vi "Main_UI_AutoPaste_2.vi"(8 "error in (no error)":errorcluster) -> (0 "error out":errorcluster)   [LabVIEW 2019]
uses:
  <vilib>/Utility/miscctls.llb/LVPointTypeDef.ctl
  <vilib>/Utility/miscctls.llb/LVPositionTypeDef.ctl
  Ctrl/Auto Inspection Main UI Ref.ctl
  Ctrl/tray icon.ctl
  Ctrl/Table Save.ctl
  Ctrl/Auto Inspection Station Name2.ctl
  Ctrl/Auto Inspection Data Name.ctl
  Function/Main UI/Glb/Main_UI Gb.vi
  Global/Process Global.vi
  LLB/Commonly VI.lvlib
panel:
  in  "NG Pick finish":bool
  in  "NG Pick arrive":bool
  in  "AI finish":bool
  in  "AI arrive":bool
  in  "LineScanfinish":bool
  in  "LineScan arrive":bool
  out "Station Name 3":string="Pick"
  in  "TrayStatus":u32[][](array[colorbox])
  in  "Tab Control":enum32{"UI", "AI  image"}(tab)
  out "Laser Station 2":string="S11 Laser Point Station"
  out "Barcode Station 2":string="S1 Barcode Station"
  out "S4 Tool String Display":string="Barcode Station"
  out "Station Name 5":string="Table4"
  out "電流":string="S4 T2 電流"
  out "電壓":string="S2 T1 電壓"
  out "Laser Station":string="Laser Point Station"
  out "Station Name 4":string="Table3"
  out "Station Name 1":string="Table1"
  out "Station Name 2":string="Table2"
  out "Barcode Status":string
  out "Laser Status":string
  out "T2 buffer":string
  out "Laser Data 2":string="S11雷射量測值"
  out "Laser Data":dbl
  out "T1 Current00":dbl
  out "S2 Tool String Display":string="Barcode Station"
  out "S3Tool String Display":string="Barcode Station"
  out "Boolean 2":bool
  out "Boolean 3":bool
  out "Boolean 4":bool
  out "Boolean 5":bool
  out "Boolean 6":bool
  out "Boolean 7":bool
  out "S2Initial":bool
  out "S2Format":bool
  out "S2Program":bool
  out "S2Scan":bool
  out "S2Reset":bool
  out "S2 T1":bool
  out "S3Initial":bool
  out "S3Format":bool
  out "S3Program":bool
  out "S3Scan":bool
  out "S3Reset":bool
  out "S3 T":bool
  out "S4Initial":bool
  out "S4Format":bool
  out "S4Program":bool
  out "S4Scan":bool
  out "S4Reset":bool
  out "S4 T":bool
  out "Total Table 2":cluster{"Table Control":string[][]}[](array[cluster])
  out "EnfMeasureTable":cluster{"Table Control":string[][]}[](array[cluster])
  out "Vision AI Status":string
  out "S8 Vision AI":string="S8 Vision AI"
  out "Barcode Action":string="Barcode Action"
  out "Vision AI":string="Barcode Action"
  out "Image 2":T1(plugin-control)
  out "image":T1(plugin-control)
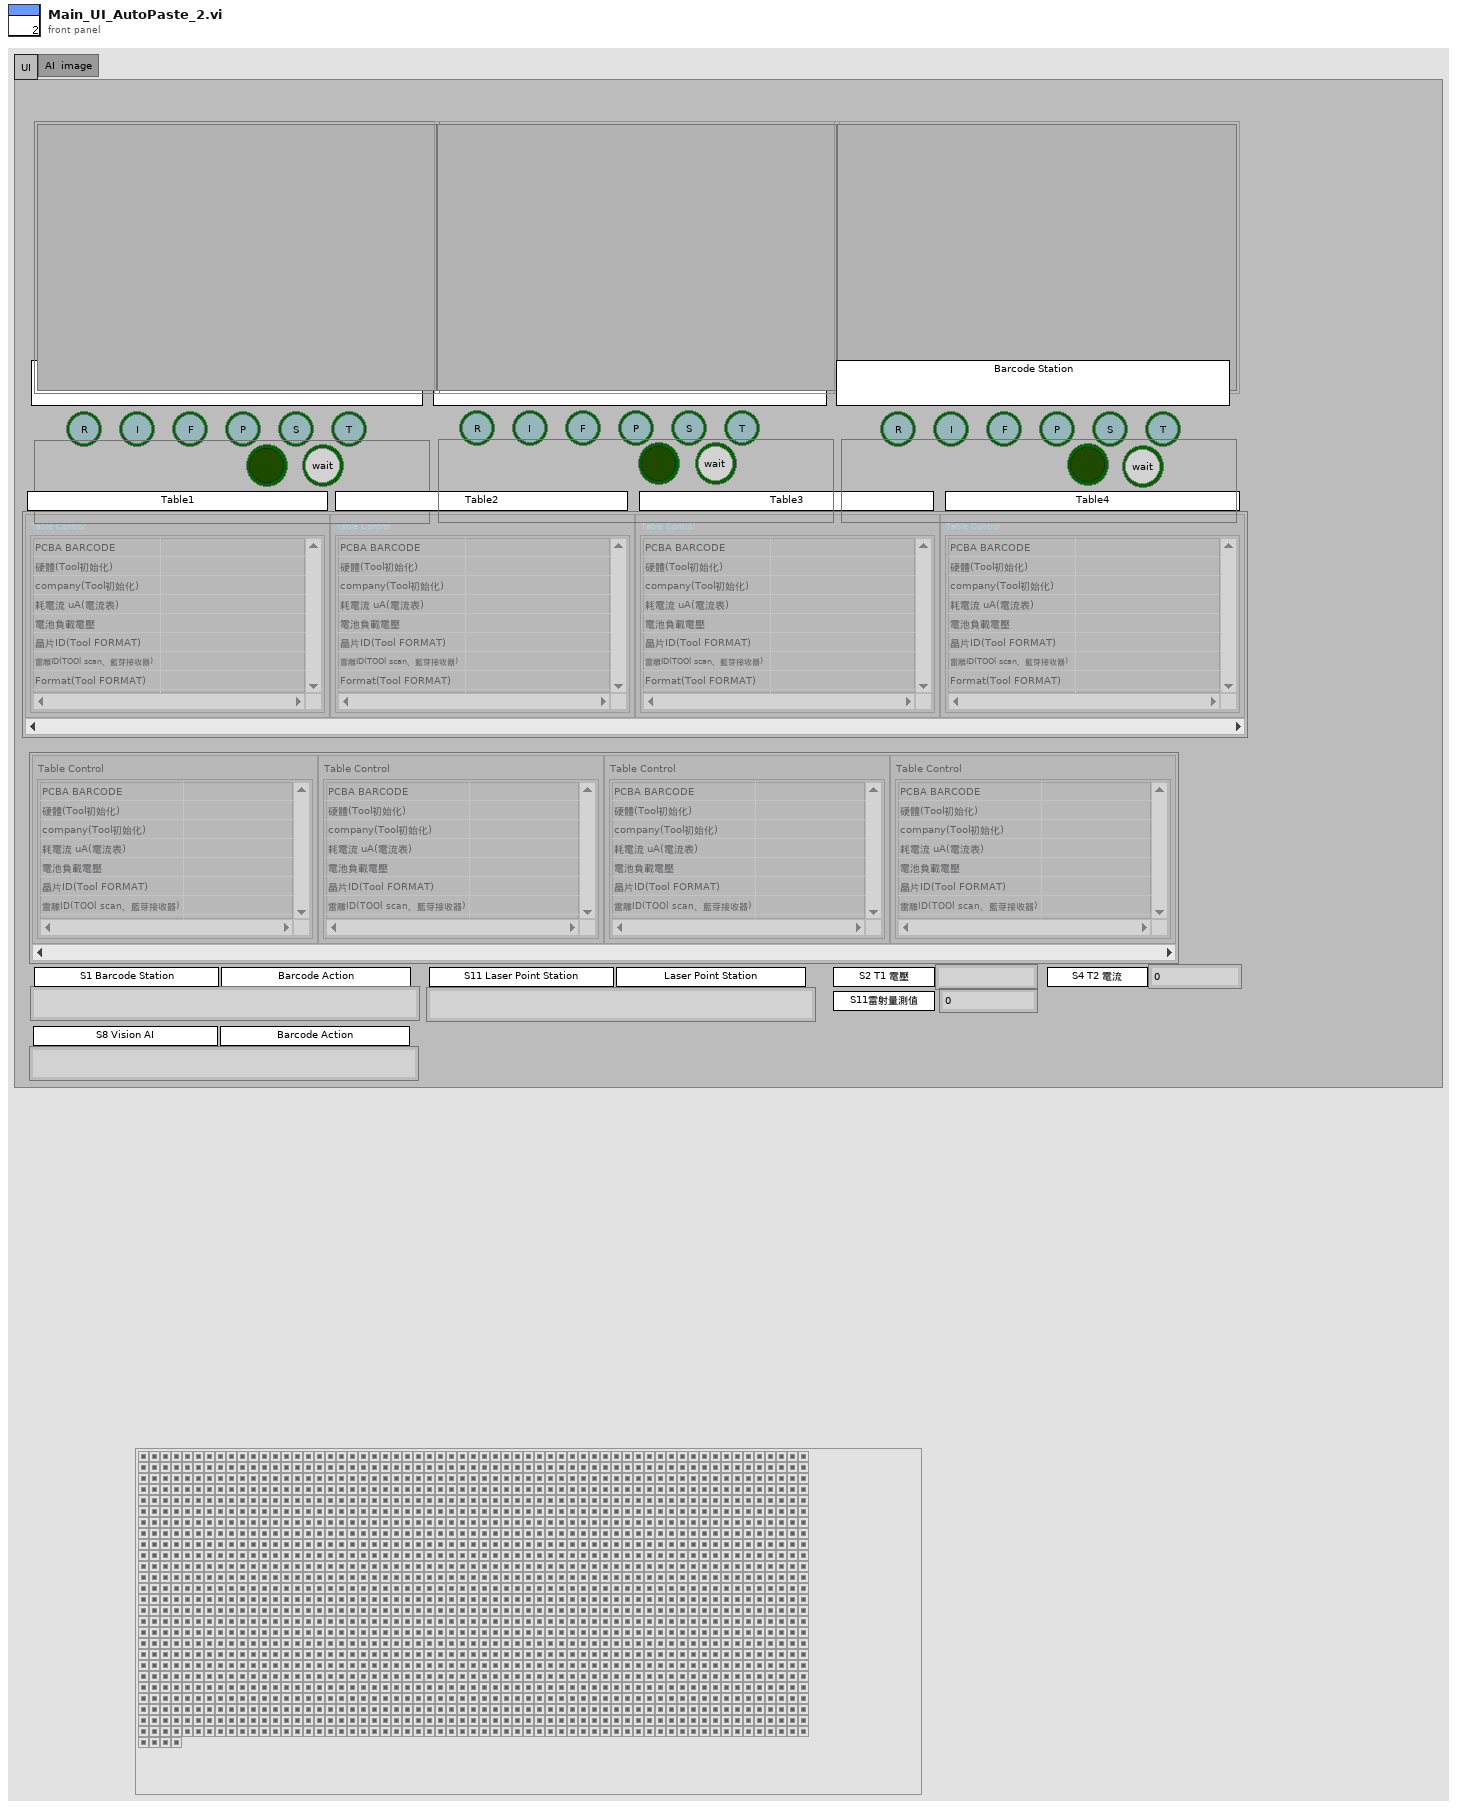
[diagram p1: front panel]
types:
  T1 = typedef "IMAQ Image.ctl" = refnum<image>
  T2 = typedef "Auto Inspection Main UI Ref.ctl" = cluster{"LineScan arrive":refnum<vi>, "LineScanfinish":refnum<vi>, "AI arrive":refnum<vi>, "AI finish":refnum<vi>, "NG Pick arrive":refnum<vi>, "NG Pick finish":refnum<vi>}
  T3 = typedef "LVPositionTypeDef.ctl" = cluster{"Left":i32, "Top":i32}
  T4 = typedef "LVPointTypeDef.ctl" = cluster{"Horizontal":i16, "Vertical":i16}
  T5 = typedef "tray icon.ctl" = u16
  T6 = typedef "Auto Inspection Data Name.ctl" = enum16{"LocalRun", "ItemSN(TimeCode)", "CurrentAction", "Error", "Data", "OKNG", "電壓值", "電壓值判斷", "電流值", "電流值判斷", "Laser1 Data", "Laser2 Data", "Laser OKNG", "StationNO"}
  T7 = typedef "Auto Inspection Station Name2.ctl" = enum16{"S1Barcode", "S2Measure", "S3Measure", "S4Measure", "S5Measure", "S11_LaserCheck", "S8_Vision AI"}
  T8 = typedef "Table Save.ctl" = enum16{"initial", "Add", "Write", "Replace", "Delete", "REad", "RedTable", "Load"}
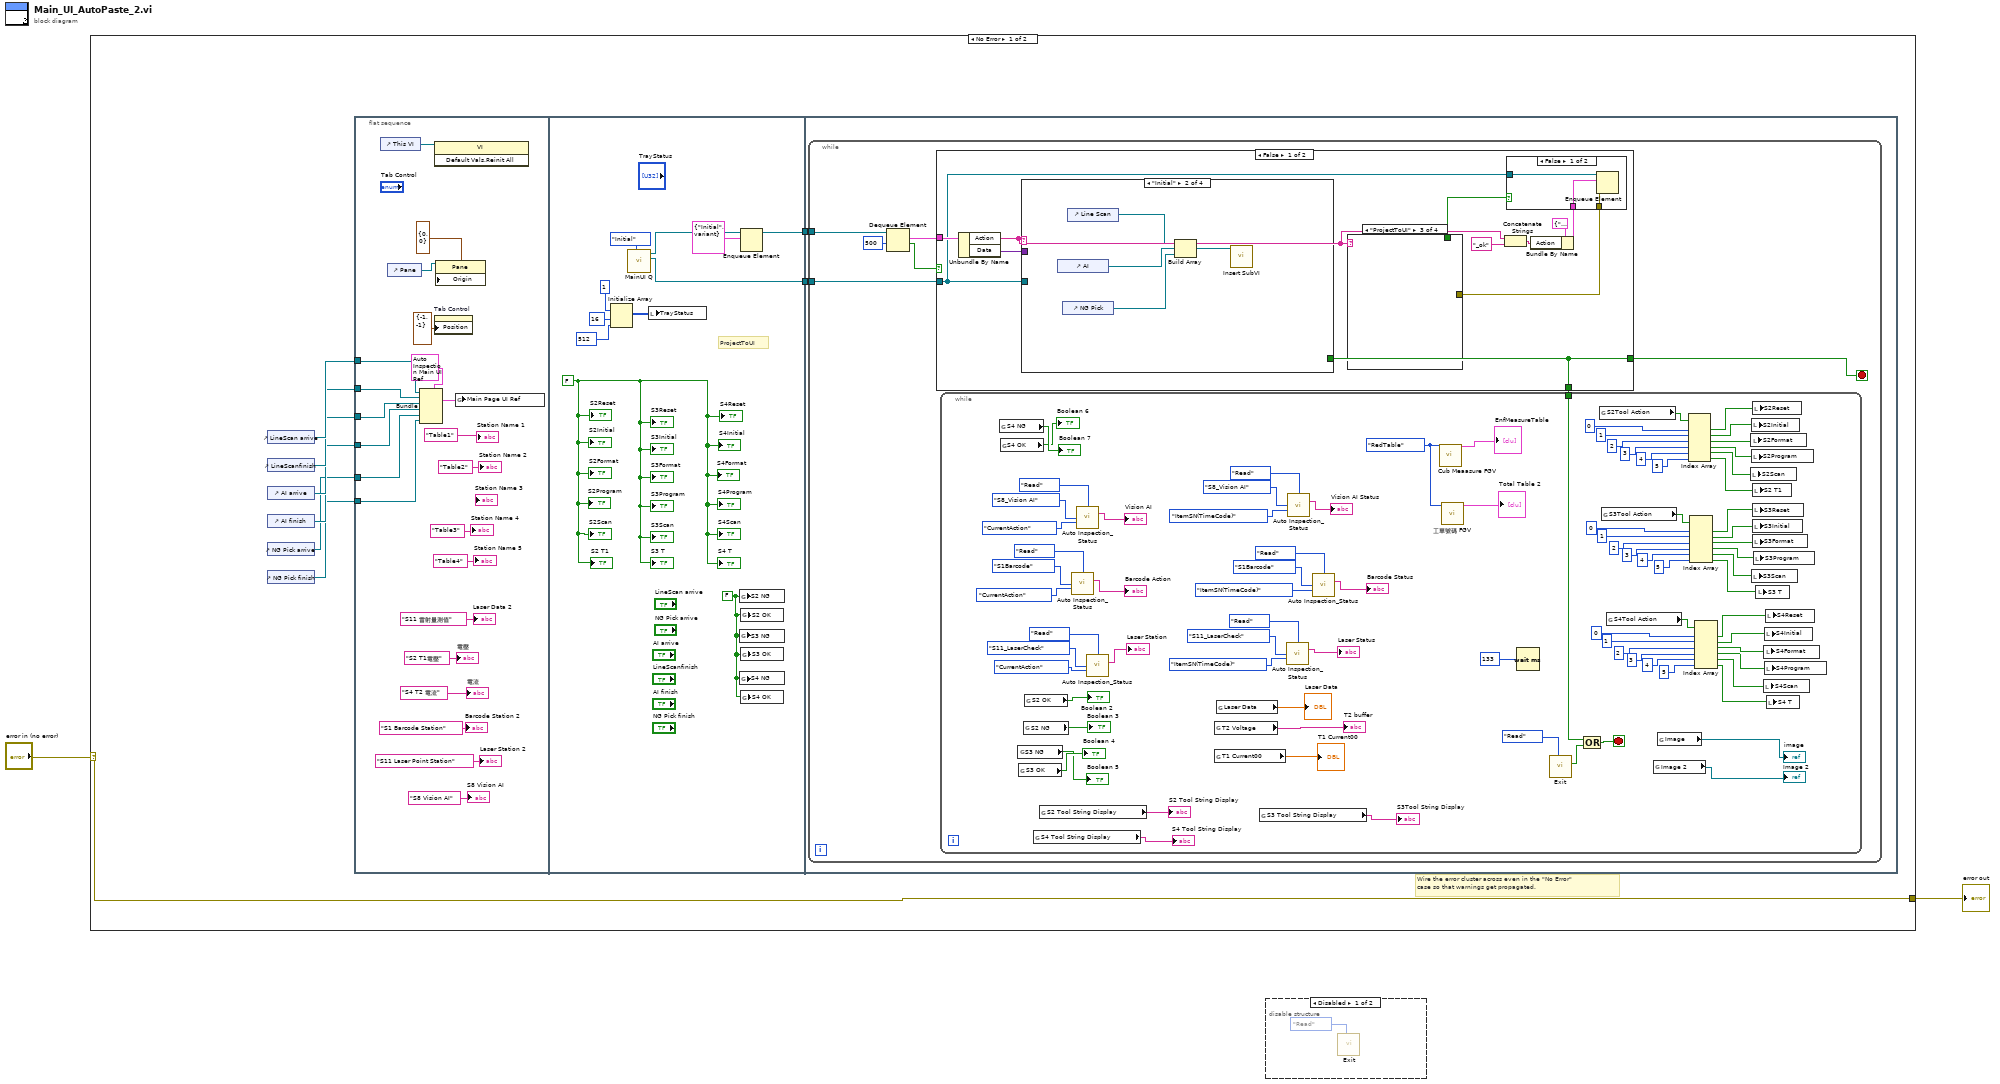
[diagram p0: block diagram]
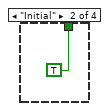
[diagram p5: hidden frame]
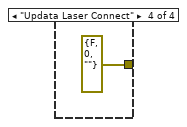
[diagram p6: hidden frame]
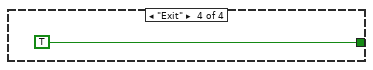
[diagram p9: hidden frame]
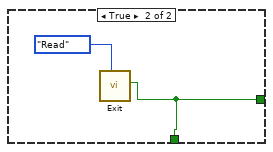
[diagram p10: hidden frame]
diagram:
  n1 = case shown="No Error" "error in (no error)" {
    selector: "error in (no error)" -> [w11 w162]
    tunnel: [w11 w162] -> w1
    frame No Error {
      # "Wire the error cluster across even in the \"No Error\"\ncase so that warnings get propagated."
      n2 = control-ref of="LineScan arrive"() -> (w8:refnum<vi>)
      n3 = control-ref of="LineScanfinish"() -> (w7:refnum<vi>)
      n4 = control-ref of="AI arrive"() -> (w6:refnum<vi>)
      n5 = control-ref of="AI finish"() -> (w5:refnum<vi>)
      n6 = control-ref of="NG Pick arrive"() -> (w4:refnum<vi>)
      n7 = control-ref of="NG Pick finish"() -> (w3:refnum<vi>)
      n8 = flat-sequence {
        tunnel: w8 -> [w28]
        tunnel: w7 -> [w27]
        tunnel: w6 -> [w26]
        tunnel: w5 -> [w25]
        tunnel: w4 -> [w24]
        tunnel: w3 -> [w23]
        tunnel: [w44] -> w10
        tunnel: [w40] -> w9
        tunnel: w10 -> [w46]
        tunnel: w9 -> [w45]
        frame #0 {
          n9 = control-ref of="This VI"() -> (w30:refnum<vi>)
          n10 = control-ref of="Pane"() -> (w33:refnum<vi>)
          n11 = Bundle(cluster=T2 {"LineScan arrive"=refnum, "LineScanfinish"=refnum, "AI arrive"=refnum, "AI finish"=refnum, "NG Pick arrive"=refnum, "NG Pick finish"=refnum}, "LineScan arrive"=w28, "LineScanfinish"=w27, "AI arrive"=w26, "AI finish"=w25, "NG Pick arrive"=w24, "NG Pick finish"=w23) -> (w29:T2)
          n12 = invoke class="VI" method="Default Vals.Reinit All"(reference=w30) -> ()  [unwired: 2 in, 3 out]
          n13 = property on="Tab Control" class="TabCtl (strict)"("Position"=T3 {"Left"=-1, "Top"=-1}) -> ()  [unwired: 2 in, 2 out]
          n14 = property class="Pane"(reference=w33, "Origin"=T4 {"Horizontal"=0, "Vertical"=0}) -> ()  [unwired: 1 in, 2 out]
          n15 = global write "Main_UI Gb.vi" "Main Page UI Ref"(w29) -> ()
          "Station Name 2" <- "Table2" ("Station Name 2")
          "Station Name 1" <- "Table1"
          "Station Name 4" <- "Table3" ("Station Name 4")
          "Laser Data 2" <- "S11 雷射量測值" ("Laser Data")
          "電壓" <- "S2 T1電壓" ("電壓")
          "電流" <- "S4 T2 電流" ("電壓")
          "Station Name 5" <- "Table4" ("Station Name 5")
          "Barcode Station 2" <- "S1 Barcode Station" ("Barcode Station 2")
          "Laser Station 2" <- "S11 Laser Point Station" ("Laser Station 2")
          "S8 Vision AI" <- "S8 Vision AI" ("S8 Vision AI")
        }
        frame #1 {
          w34 = FALSE ("S2 NG")
          w35 = FALSE ("S2 NG")
          # "ProjectToUI"
          n16 = Initialize Array(T5 1 ("Ring"), 16 ("dimension size"), 512 ("dimension size")) -> (w36:T5[][])
          n17 = call "MainUI Q.vi"("Enum"=enum16{"Initial", "read", "release"}."Initial") -> ("UI Response Out"=w40:refnum<queue>, "UI Receive Out"=w41:refnum<queue>)  [unwired: 9 in]
          n18 = local write "TrayStatus"(w36) -> ()
          n19 = global write "Process Global.vi" "S2 NG"(w35) -> ()
          n20 = global write "Process Global.vi" "S3 NG"(w35) -> ()
          n21 = global write "Process Global.vi" "S4 NG"(w35) -> ()
          n22 = Enqueue Element(queue=w41, element=cluster{"Action":string, "Data":variant} {"Action"="Initial", "Data"=variant}) -> (queue out=w44:refnum<queue>)  [unwired: 2 in, 2 out]
          n23 = global write "Process Global.vi" "S2 OK"(w35) -> ()
          n24 = global write "Process Global.vi" "S3 OK"(w35) -> ()
          n25 = global write "Process Global.vi" "S4 OK"(w35) -> ()
          "S2Initial" <- w34
          "S2Format" <- w34
          "S2Program" <- w34
          "S2Scan" <- w34
          "S2 T1" <- w34
          "S2Reset" <- w34
          "S3Reset" <- w34
          "S3Initial" <- w34
          "S3Format" <- w34
          "S3Program" <- w34
          "S3Scan" <- w34
          "S3 T" <- w34
          "S4Reset" <- w34
          "S4Format" <- w34
          "S4Initial" <- w34
          "S4Program" <- w34
          "S4Scan" <- w34
          "S4 T" <- w34
        }
        frame #2 {
          n26 = while {
            tunnel: w46 -> [w53]
            tunnel: w45 -> [w51]
            stop <- w50 stop-if-true
            n27 = Dequeue Element(queue=w53, timeout in ms (-1)=500) -> (element=w52:cluster{"Action":string, "Data":variant}, timed out?=w49:bool)  [unwired: 1 in, 2 out]
            n28 = case shown="False" w49 {
              tunnel: w52 -> [w149 _]
              tunnel: w51 -> [w147 _]
              tunnel: [w139 w160] -> w50
              tunnel: [w139 w160] -> w47
              frame False {
                n29 = Unbundle By Name(w149) -> ("Action"=w143:string, "Data"=w148:variant)
                n30 = case shown="\"Initial\"" w143 {
                  tunnel: w147 -> [_ _ _ _]
                  tunnel: [_ _ _ TRUE] -> w139
                  tunnel: w148 -> [_ _ _ _]
                  frame "False", Default {
                  }
                  frame "Initial" {
                    n31 = control-ref of="AI"() -> (w157:refnum<vi>)
                    n32 = control-ref of="NG Pick"() -> (w156:refnum<vi>)
                    n33 = control-ref of="Line Scan"() -> (w158:refnum<vi>)
                    n34 = Build Array(w158, w157, w156) -> (w155:refnum<vi>[])
                    n35 = call "Insert SubVI.vi"("Sub UI"=w155) -> ()  [unwired: 11 in]
                  }
                  frame "SetSyms" {
                  }
                  frame "Exit" {
                  }
                }
                n36 = case shown="\"ProjectToUI\"" w143 {
                  tunnel: [_ _ _ errorcluster {"status"=FALSE, "code"=0, "source"=""} ("error constant")] -> w141
                  tunnel: [_ TRUE _ _] -> w140
                  frame "False", Default {
                  }
                  frame "Initial" {
                  }
                  frame "ProjectToUI" {
                  }
                  frame "Updata Laser Connect" {
                  }
                }
                n37 = Concatenate Strings(w143, "_ok" ("string")) -> (w144:string)
                n38 = Bundle By Name(cluster=cluster{"Action":string, "Data":variant} {"Action"="", "Data"=variant} ("element"), "Action"=w144) -> (w145:cluster{"Action":string, "Data":variant})
                n39 = case shown="False" w140 {
                  tunnel: w147 -> [w152 _]
                  tunnel: w145 -> [w151 _]
                  tunnel: w141 -> [w150 _]
                  frame False {
                    n40 = Enqueue Element(queue=w152, element=w151, error in (no error)=w150) -> ()  [unwired: 1 in, 3 out]
                  }
                  frame True {
                  }
                }
              }
              frame True {
                n41 = call "Exit.vi"("Enum"=enum16{"Initial", "Read", "Write"}."Read") -> ("ExitOut"=w160:bool)  [unwired: 10 in]
              }
            }
            n42 = while {
              tunnel: w47 -> [w124]
              stop <- w122 stop-if-true
              w68 = Table_Save."RedTable" ("Enum")
              n43 = global read "Process Global.vi" "S4 NG"() -> (→"Boolean 7":bool)
              n44 = global read "Process Global.vi" "S4 OK"() -> (→"Boolean 6":bool)
              n45 = global read "Process Global.vi" "S3 NG"() -> (→"Boolean 5":bool)
              n46 = global read "Process Global.vi" "S3 OK"() -> (→"Boolean 4":bool)
              n47 = global read "Process Global.vi" "S2 NG"() -> (→"Boolean 3":bool)
              n48 = global read "Process Global.vi" "S2 OK"() -> (→"Boolean 2":bool)
              n49 = global read "Process Global.vi" "S4 Tool String Display"() -> (→"S4 Tool String Display":string)
              n50 = global read "Process Global.vi" "S2 Tool String Display"() -> (→"S2 Tool String Display":string)
              n51 = call "Auto Inspection_Status.vi"("Action"=enum16{"Initial", "Write", "Read"}."Read", "Station"=Auto_Inspection_Station_Name2."S1Barcode", "Data"=Auto_Inspection_Data_Name."CurrentAction") -> ("DataOut"=→"Barcode Action":string)  [unwired: 10 in, 2 out]
              n52 = call "Auto Inspection_Status.vi"("Action"=enum16{"Initial", "Write", "Read"}."Read", "Station"=Auto_Inspection_Station_Name2."S8_Vision AI", "Data"=Auto_Inspection_Data_Name."CurrentAction") -> ("DataOut"=→"Vision AI":string)  [unwired: 10 in, 2 out]
              n53 = call "Auto Inspection_Status.vi"("Action"=enum16{"Initial", "Write", "Read"}."Read", "Station"=Auto_Inspection_Station_Name2."S11_LaserCheck", "Data"=Auto_Inspection_Data_Name."CurrentAction") -> ("DataOut"=→"Laser Station":string)  [unwired: 10 in, 2 out]
              n54 = global read "Process Global.vi" "T2 Voltage"() -> (→"T2 buffer":string)
              n55 = global read "Process Global.vi" "T1 Current00"() -> (→"T1 Current00":dbl)
              n56 = global read "Process Global.vi" "Laser Data"() -> (→"Laser Data":dbl)
              n57 = global read "Process Global.vi" "S3 Tool String Display"() -> (→"S3Tool String Display":string)
              n58 = call "Auto Inspection_Status.vi"("Action"=enum16{"Initial", "Write", "Read"}."Read", "Station"=Auto_Inspection_Station_Name2."S11_LaserCheck", "Data"=Auto_Inspection_Data_Name."ItemSN(TimeCode)") -> ("DataOut"=→"Laser Status":string)  [unwired: 10 in, 2 out]
              n59 = call "Auto Inspection_Status.vi"("Action"=enum16{"Initial", "Write", "Read"}."Read", "Station"=Auto_Inspection_Station_Name2."S8_Vision AI", "Data"=Auto_Inspection_Data_Name."ItemSN(TimeCode)") -> ("DataOut"=→"Vision AI Status":string)  [unwired: 10 in, 2 out]
              n60 = call "Auto Inspection_Status.vi"("Action"=enum16{"Initial", "Write", "Read"}."Read", "Station"=Auto_Inspection_Station_Name2."S1Barcode", "Data"=Auto_Inspection_Data_Name."ItemSN(TimeCode)") -> ("DataOut"=→"Barcode Status":string)  [unwired: 10 in, 2 out]
              n61 = call "Cub Meaasure FGV.vi"("Action"=w68) -> ("Total Table"=→"EnfMeasureTable":cluster{"Table Control":string[][]}[])  [unwired: 11 in, 7 out]
              n62 = call "工單號碼 FGV.vi"("Action"=w68) -> ("Total Table"=→"Total Table 2":cluster{"Table Control":string[][]}[])  [unwired: 11 in, 7 out]
              n63 = Wait (ms)(milliseconds to wait=133) -> ()  [unwired: 1 out]
              n64 = call "Exit.vi"("Enum"=enum16{"Initial", "Read", "Write"}."Read") -> ("ExitOut"=w123:bool)  [unwired: 10 in]
              n65 = Compound Arithmetic op=OR(w124, w123) -> (w122:bool)
              n66 = global read "Process Global.vi" "S2Tool Action"() -> (w114:bool[])
              n67 = global read "Process Global.vi" "S3Tool Action"() -> (w89:bool[])
              n68 = global read "Process Global.vi" "S4Tool Action"() -> (w88:bool[])
              n69 = global read "Process Global.vi" "Image 2"() -> (→"Image 2":T1)
              n70 = global read "Process Global.vi" "Image"() -> (→"image":T1)
              n71 = Index Array(array=w114, index #1=0 ("index"), index #2=1 ("index"), index #3=2 ("index"), index #4=3 ("index"), index #5=4 ("index"), index #6=5 ("index")) -> (element #1=w107:bool, element #2=w106:bool, element #3=w105:bool, element #4=w104:bool, element #5=w103:bool, element #6=w102:bool)
              n72 = Index Array(array=w89, index #1=0 ("index"), index #2=1 ("index"), index #3=2 ("index"), index #4=3 ("index"), index #5=4 ("index"), index #6=5 ("index")) -> (element #1=w96:bool, element #2=w97:bool, element #3=w98:bool, element #4=w99:bool, element #5=w100:bool, element #6=w101:bool)
              n73 = Index Array(array=w88, index #1=0 ("index"), index #2=1 ("index"), index #3=2 ("index"), index #4=3 ("index"), index #5=4 ("index"), index #6=5 ("index")) -> (element #1=w81:bool, element #2=w80:bool, element #3=w79:bool, element #4=w78:bool, element #5=w77:bool, element #6=w76:bool)
              n74 = local write "S2Scan"(w103) -> ()
              n75 = local write "S2Format"(w105) -> ()
              n76 = local write "S2Initial"(w106) -> ()
              n77 = local write "S2Program"(w104) -> ()
              n78 = local write "S3Scan"(w100) -> ()
              n79 = local write "S2Reset"(w107) -> ()
              n80 = local write "S2 T1"(w102) -> ()
              n81 = local write "S3Reset"(w96) -> ()
              n82 = local write "S3Initial"(w97) -> ()
              n83 = local write "S3Format"(w98) -> ()
              n84 = local write "S3Program"(w99) -> ()
              n85 = local write "S3 T"(w101) -> ()
              n86 = local write "S4Scan"(w77) -> ()
              n87 = local write "S4Format"(w79) -> ()
              n88 = local write "S4Initial"(w80) -> ()
              n89 = local write "S4Program"(w78) -> ()
              n90 = local write "S4Reset"(w81) -> ()
              n91 = local write "S4 T"(w76) -> ()
            }
          }
        }
      }
    }
    frame Error {
    }
  }
  "error out" <- w1
  n92 = disable-structure shown="Disabled" {
    frame Disabled {
      n93 = call "Exit.vi"("Enum"=enum16{"Initial", "Read", "Write"}."Read") -> ()  [unwired: 10 in, 1 out]
    }
    frame Enabled {
    }
  }
